vi "GetPathFromName.vi"(4 "Experience ID":string="TestOK\nTest") -> (0 "VI_Path":path, 1 "application reference":refnum<vi>, 2 "Error out":errorcluster={"status"=TRUE, "code"=2, "source"="incorrect path for Experience ID"})   [LabVIEW 2020]
uses:
  Configuration/Global_Configurations.vi
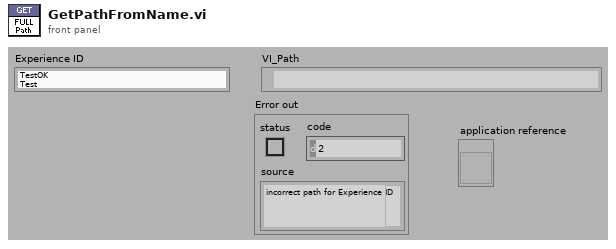
[diagram p1: front panel]
types:
  T1 = cluster{"LabVIEW Host":string, "LabVIEW Port":u16, "Path":path, "Name":string, "Authors":string, "Keywords":string, "Description":string, "Cameras":cluster{"Base URL":string, "Path":string, "Name":string}[], "Sampling":cluster{"Sampled Variable":string, "Delta":dbl}[], "Sampling Freq":u32}[]
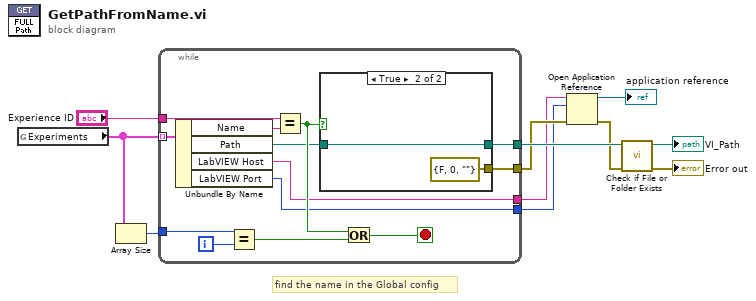
[diagram p0: block diagram]
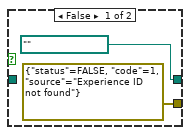
[diagram p2: hidden frame]
diagram:
  # "find the name in the Global config"
  n1 = global read "Global_Configurations.vi" "Experiments"() -> (w11:T1)
  n2 = Array Size(array=w11) -> (size(s)=w10:i32)
  n3 = while {
    tunnel: w11 -> [w24] mode=indexing
    tunnel: "Experience ID" -> [w23]
    tunnel: w10 -> [w21]
    tunnel: [w17] -> w8
    tunnel: [w15] -> w4
    tunnel: [w13] -> w2
    tunnel: [w12] -> w1
    i -> [w22]
    stop <- w19 stop-if-true
    n4 = Unbundle By Name(w24) -> ("Name"=w20:string, "Path"=w14:path, "LabVIEW Host"=w13:string, "LabVIEW Port"=w12:u16)
    n5 = Equal?(x=w21, y=w22) -> (x = y?=w18:bool)
    n6 = Equal?(x=w23, y=w20) -> (x = y?=w16:bool)
    n7 = case shown="True" w16 {
      tunnel: w14 -> [_ w28]
      tunnel: [path "" ("Path") w28] -> w17
      tunnel: [errorcluster {"status"=FALSE, "code"=1, "source"="Experience ID not found"} ("error in (no error)") errorcluster {"status"=FALSE, "code"=0, "source"=""} ("error in (no error)")] -> w15
      frame False {
      }
      frame True {
      }
    }
    n8 = Or(x=w16, y=w18) -> (x .or. y?=w19:bool)
  }
  n9 = Open Application Reference(8:w4, 10:w1, 11:w2) -> (0:w3:errorcluster, 3:→"application reference":refnum<vi>)  [unwired: 1 in]
  n10 = call <vilib>:"Check if File or Folder Exists.vi"("error in (no error)"=w3, "path"=w8) -> ("error out"=→"Error out":errorcluster, "dup path"=→"VI_Path":path)  [unwired: 8 out]
